vi "PWM Driver Calibration Popup.vi"(8 "error in (no error)":errorcluster, 10 "Message":string="The PWM stimulus parameters have been set, but the PWM requires calibration and zeroing.\n\nPlease perform the following steps:\n\n1)  Connect the Power Sensor to the Power Ref port;\n2)  Press Calibrate.", 11 "Header":string="Normalization of the Agilent E4418B PWM") -> (0 "error out":errorcluster, 3 "Dialog Response":string)   [LabVIEW 2011]
panel:
  in  "Cancel":bool
  in  "Calibrate":bool
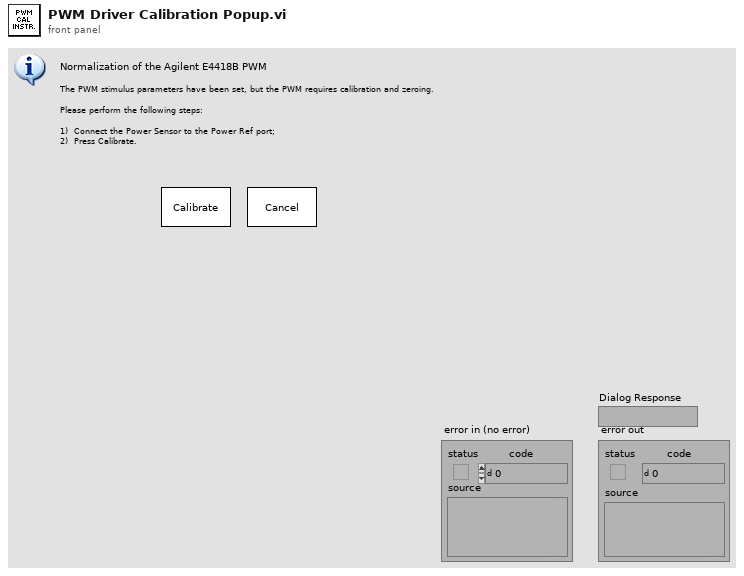
[diagram p1: front panel]
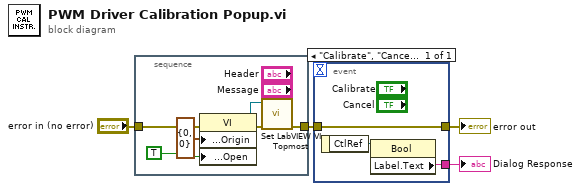
[diagram p0: block diagram]
diagram:
  n1 = stacked-sequence {
    tunnel: "error in (no error)" -> [w10]
    tunnel: [w7] -> w2
    frame #0 {
      n2 = property on="Property Node" class="VI"(error in=w10, "Front Panel Window:Origin"=cluster{"Horizontal":i16, "Vertical":i16} {"Horizontal"=0, "Vertical"=0}, "Front Panel Window:Open"=TRUE) -> (reference out=w6:refnum<vi>, error out=w8:errorcluster)  [unwired: 1 in]
      n3 = call "Set LabVIEW VI Topmost.vi"("error in (no error)"=w8, "VI Refnum (null)"=w6) -> ("error out"=w7:errorcluster)  [unwired: 7 in, 2 out]
    }
  }
  n4 = event shown="[0] \"Calibrate\", \"Cancel\": Value Change" {
    selector: _ -> [_]
    dyn-events: _ -> [_]
    timeout: _ -> [_]
    tunnel: w2 -> [w13]
    tunnel: [w13] -> w4
    tunnel: [w11] -> w1
    event "Calibrate", "Cancel": Value Change {
      n5 = event-data() -> ("CtlRef"=w12:refnum<vi>)  [unwired: 1 out]
      n6 = property on="Property Node" class="Bool"(reference=w12) -> ("Label.Text"=w11:string)  [unwired: 1 in, 2 out]
    }
  }
  "error out" <- w4
  "Dialog Response" <- w1
